vi "TEST - Read INI Cluster.vi"(8 "error in (no error)":errorcluster) -> (0 "error out":errorcluster, 2 "Passed":bool)   [LabVIEW 2020]
uses:
  <vilib>/addons/_JKI Toolkits/Caraya/classes/Assert/Assert True.vi
  <vilib>/Utility/config.llb/NI_LVConfig.lvlib
  <userlib>/_OpenG.lib/file/file.llb/openg_file.lvlib
  <vilib>/addons/_JKI Toolkits/Caraya/classes/Test/Test.lvclass
  <vilib>/addons/_JKI Toolkits/Caraya/classes/Assert/Assert.lvclass
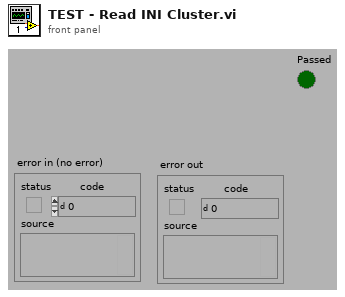
[diagram p1: front panel]
types:
  T1 = cluster{"Section 1":cluster{"Float":dbl, "Integer":i32}, "Section 2":cluster{"Boolean":bool, "String":string}}
  T2 = typedef "NI_LVConfig.lvlib/Config Data RefNum.ctl" = refnum<k1>
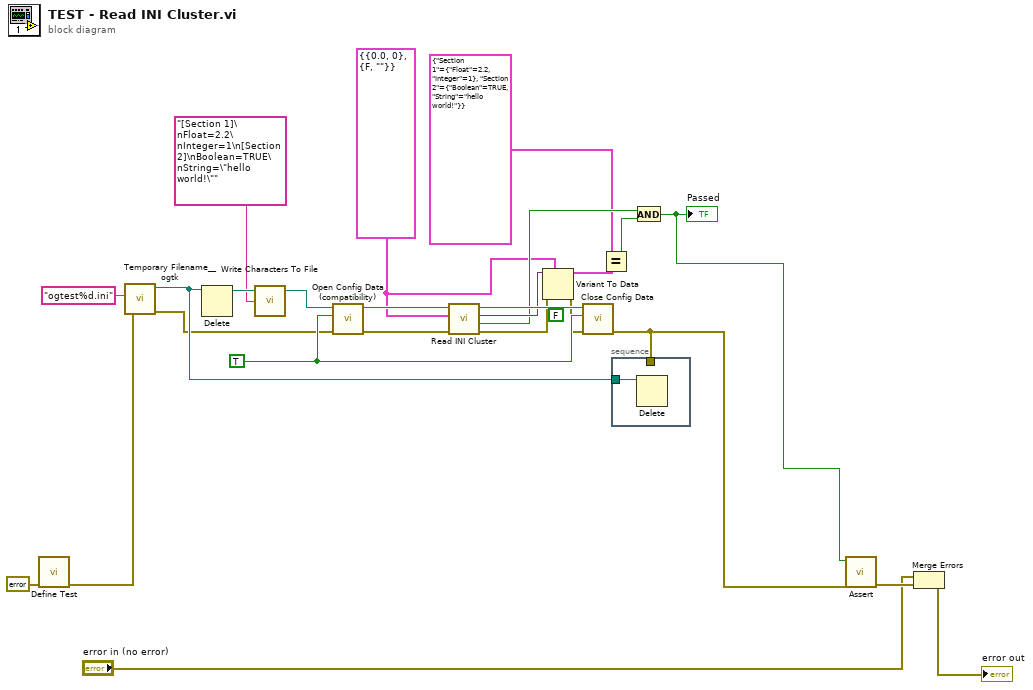
[diagram p0: block diagram]
diagram:
  (unwired) FALSE ("write configuration file? (T)")
  w12 = T1 {"Section 1"={"Float"=0.0, "Integer"=0}, "Section 2"={"Boolean"=FALSE, "String"=""}}
  w24 = TRUE ("create file if necessary? (T)")
  n1 = call <vilib>:"Define Test.vi"("error in (no error)"=errorcluster {"status"=FALSE, "code"=0, "source"=""}) -> ("error out"=w6:errorcluster)  [unwired: 9 in, 1 out]
  n2 = call <userlib>:"Temporary Filename__ogtk.vi"("error in (no error)"=w6, "pattern (lvtemp%d.tmp)"="ogtest%d.ini") -> ("error out"=w8:errorcluster, "file in tmp dir"=w10:path)  [unwired: 4 in]
  n3 = Delete(path (use dialog)=w10) -> (deleted path=w17:path)  [unwired: 4 in, 2 out]
  n4 = call <vilib>:"Write Characters To File.vi"("character string"="[Section 1]\nFloat=2.2\nInteger=1\n[Section 2]\nBoolean=TRUE\nString=\"hello world!\"", "file path (dialog if empty)"=w17) -> ("new file path (Not A Path if cancelled)"=w16:path)  [unwired: 3 in]
  n5 = call <vilib>:"Open Config Data (compatibility).vi"("error in (no error)"=w8, "create file if necessary (T)"=w24, "configuration file path"=w16) -> ("error out"=w13:errorcluster, "refnum"=w14:T2)  [unwired: 6 in, 1 out]
  n6 = call "Read INI Cluster.vi"("error in (no error)"=w13, "INI Fomatted Cluster Type"=w12, "refnum"=w14) -> ("error out"=w21:errorcluster, "all found?"=w19:bool, "INI Fomatted Cluster"=w23:variant, "dup refnum"=w25:T2)  [unwired: 4 in, 1 out]
  n7 = Variant To Data(error in=w21, type=w12, Variant=w23) -> (data=w18:T1, error out=w22:errorcluster)
  n8 = call <vilib>:"Close Config Data.vi"("error in (no error)"=w22, "write file if changed (T)"=w24, "refnum"=w25) -> ("error out"=w5:errorcluster)  [unwired: 7 in, 1 out]
  n9 = Equal?(x=T1 {"Section 1"={"Float"=2.2, "Integer"=1}, "Section 2"={"Boolean"=TRUE, "String"="hello world!"}}, y=w18) -> (x = y?=w20:bool)
  n10 = stacked-sequence {
    tunnel: w10 -> [w26]
    tunnel: w5 -> [_]
    frame #0 {
      n11 = Delete(path (use dialog)=w26) -> ()  [unwired: 4 in, 3 out]
    }
  }
  n12 = And(x=w19, y=w20) -> (x .and. y?=w2:bool)
  "Passed" <- w2
  n13 = call-poly <vilib>:"Assert.vi"("error in (no error)"=w5, "True?"=w2) -> ("error out"=w7:errorcluster)  [unwired: 8 in, 1 out]
  n14 = Merge Errors("error in (no error)", w7) -> (→"error out":errorcluster)
